vi "Get Description.vi"(8 "error in (no error)":errorcluster, 11 "Housekeeping in":refnum<class "Housekeeping.lvclass">) -> (0 "error out":errorcluster, 2 "Service Description":string, 3 "Housekeeping out":refnum<class "Housekeeping.lvclass">)   [LabVIEW 2023, in "Room Service Types.lvlib" / "Housekeeping.lvclass"]
uses:
  Housekeeping.lvclass
  Housekeeping.lvclass/Housekeeping.ctl
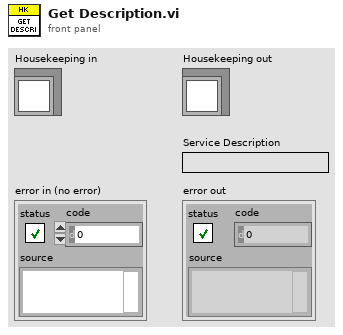
[diagram p1: front panel]
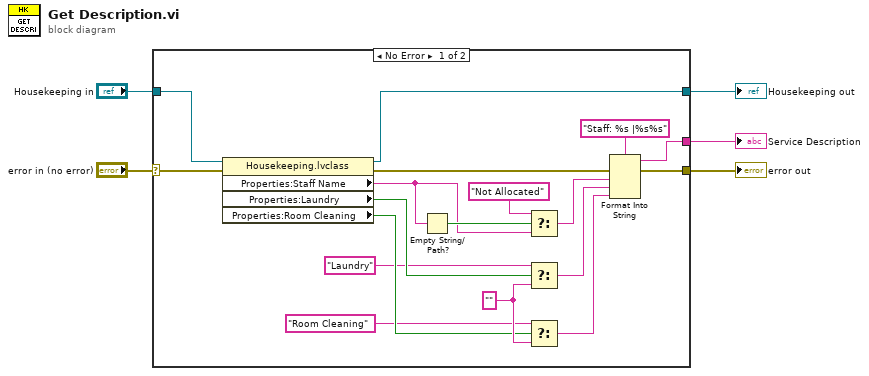
[diagram p0: block diagram]
diagram:
  n1 = case shown="No Error" "error in (no error)" {
    selector: "error in (no error)" -> [w23 w24]
    tunnel: [w22 w24] -> w4
    tunnel: "Housekeeping in" -> [w20 w25]
    tunnel: [w19 w25] -> w2
    tunnel: [w18 _] -> w1
    frame No Error {
      w13 = "" ("format string")
      n2 = property class="Housekeeping.lvclass"(reference=w20, error in=w23) -> (reference out=w19:refnum<class "Housekeeping.lvclass">, error out=w21:errorcluster, "Properties:Staff Name"=w14:string, "Properties:Laundry"=w12:bool, "Properties:Room Cleaning"=w11:bool)
      n3 = Empty String/Path?(string/path=w14) -> (empty?=w16:bool)
      n4 = Select(t="Not Allocated" ("format string"), s=w16, f=w14) -> (s? t:f=w6:string)
      n5 = Select(t="Laundry" ("format string"), s=w12, f=w13) -> (s? t:f=w7:string)
      n6 = Select(t="Room Cleaning" ("format string"), s=w11, f=w13) -> (s? t:f=w8:string)
      n7 = Format Into String(format string="Staff: %s |%s%s", error in=w21, w6, w7, w8) -> (resulting string=w18:string, error out=w22:errorcluster)  [unwired: 1 in]
    }
    frame Error {
    }
  }
  "error out" <- w4
  "Housekeeping out" <- w2
  "Service Description" <- w1
